vi "Start tasks.vi"(8 "error in (no error)":errorcluster, 10 "Device model":string, 11 "Module ID":i32=-1) -> (0 "error out":errorcluster)   [LabVIEW 2020]
doc: "Start all tasks, except CI task. Set all outputs to initial values."
uses:
  NI_DAQ/Libraries/NI DAQ/NI DAQ.lvlib
  NI_DAQ/Libraries/NI DAQ/Support/Task list.ctl
  controls/Motor FGV states ---typedef.ctl
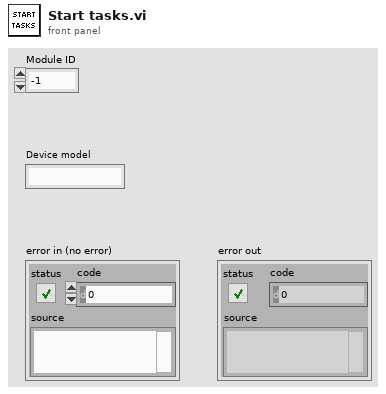
[diagram p1: front panel]
types:
  T1 = typedef "Motor FGV states ---typedef.ctl" = enum16{"Set", "Reset", "Get"}
  T2 = typedef "NI DAQ.lvlib/Task list.ctl" = enum16{"All", "DO task", "DI task", "AO task", "AI task", "CI task", "CO task", "TC task"}
  T3 = typedef "Motor controls---typedef.ctl" = cluster{"EN1":bool, "DIR1":bool, "EN2":bool, "DIR2":bool, "TOG":bool}
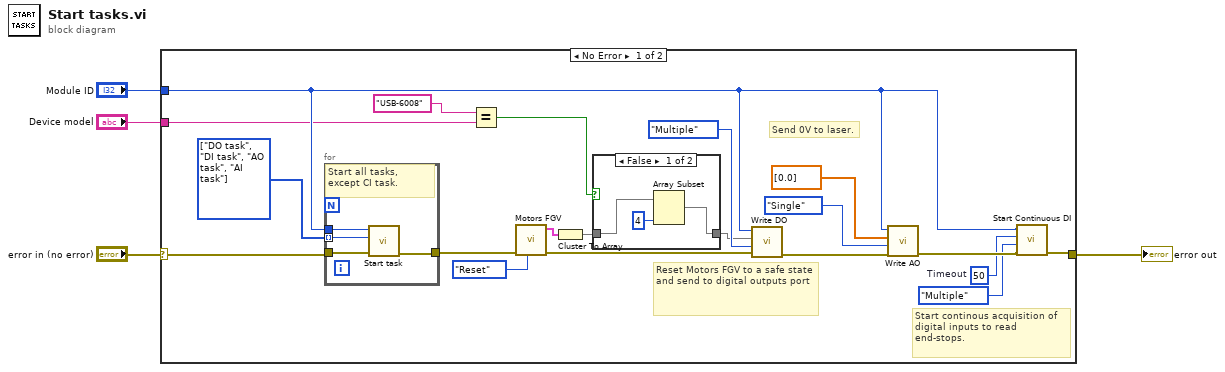
[diagram p0: block diagram]
diagram:
  n1 = case shown="No Error" "error in (no error)" {
    selector: "error in (no error)" -> [w23 w33]
    tunnel: "Module ID" -> [w10 _]
    tunnel: [w14 w33] -> w2
    tunnel: "Device model" -> [w9 _]
    frame No Error {
      w12 = 50  # Timeout
      w22 = T2[] [enum."DO task", enum."DI task", enum."AO task", enum."AI task"] items=["All", "DO task", "DI task", "AO task", "AI task", "CI task", "CO task", "TC task"] ("Array")
      # "Start continous acquisition of digital inputs to read end-stops."
      # "Reset Motors FGV to a safe state and send to digital outputs port"
      # "Send 0V to laser."
      n2 = for {
        tunnel: w10 -> [w30]
        tunnel: w22 -> [w29] mode=indexing
        tunnel: w23 -> [w32]
        tunnel: [w31] -> w18
        # "Start all tasks, except CI task."
        n3 = call "Start task.vi"("error in"=w32, "Task list"=w29, "Module ID"=w30) -> ("error out"=w31:errorcluster)  [unwired: 8 in]
      }
      n4 = Equal?(x="USB-6008", y=w9) -> (x = y?=w7:bool)
      n5 = call "Motors FGV.vi"("Action"=Motor_FGV_states_---typedef."Reset", "error in (no error)"=w18) -> ("error out"=w17:errorcluster, "Motor control out"=w16:T3)  [unwired: 8 in]
      n6 = Cluster To Array(cluster=w16) -> (array=w6:bool[])
      n7 = case shown="False" w7 {
        tunnel: w6 -> [w27 w28]
        tunnel: [w25 w28] -> w5
        frame False {
          n8 = Array Subset(array=w27, length=4) -> (w25:bool[])  [unwired: 1 in]
        }
        frame True {
        }
      }
      n9 = call "Write DO.vi"("error in"=w17, "Samples"=enum16{"Single", "Multiple"}."Multiple", "Data"=w5, "Module ID"=w10) -> ("error out"=w21:errorcluster)  [unwired: 7 in]
      n10 = call "Write AO.vi"("error in"=w21, "Samples"=enum16{"Single", "Multiple"}."Single", "Value(s)"=dbl[] [0.0], "Module ID"=w10) -> ("error out"=w13:errorcluster)  [unwired: 7 in]
      n11 = call "Start Continuous DI.vi"("error in"=w13, "Acq type"=enum16{"Single", "Multiple"}."Multiple", "Timeout"=w12, "Module ID"=w10) -> ("error out"=w14:errorcluster)  [unwired: 7 in]
    }
    frame Error {
    }
  }
  "error out" <- w2
